vi "Splitter Manager UI.vi"(8 "error in (no error)":errorcluster, 11 "QD VI":refnum<vi>) -> (0 "error out":errorcluster)   [LabVIEW 2017]
uses:
  Splitter Info.ctl
panel:
  in  "Type Selector":enum32{"Splitters", "Panes"}(radio) caption="Radio Buttons"
  in  "Splitters":T1[](array[typedef])
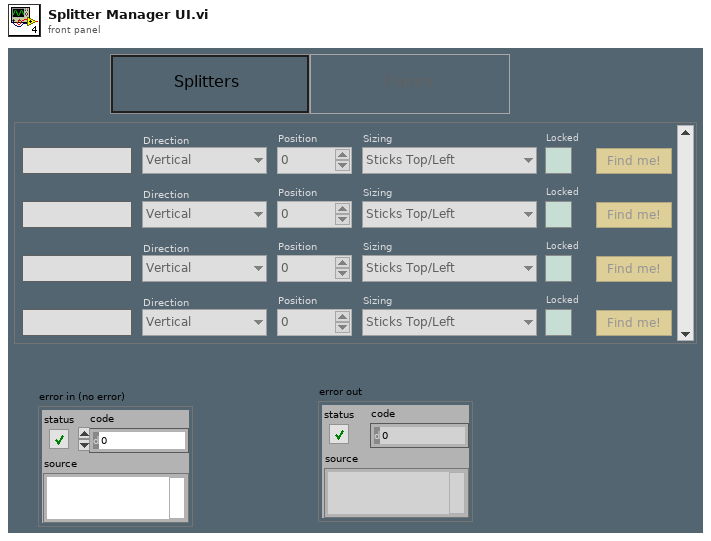
[diagram p1: front panel]
types:
  T1 = typedef "Splitter Info.ctl" = cluster{"Label":string, "Position":i32, "Sizing":enum16{"Sticks Top/Left", "Sticks Bottom/Right", "Proportional"}, "Locked":bool, "Highlight":bool, "Direction":enum16{"Vertical", "Horizontal"}}
  T2 = enum16{"Sticks Top/Left", "Sticks Bottom/Right", "Proportional"}
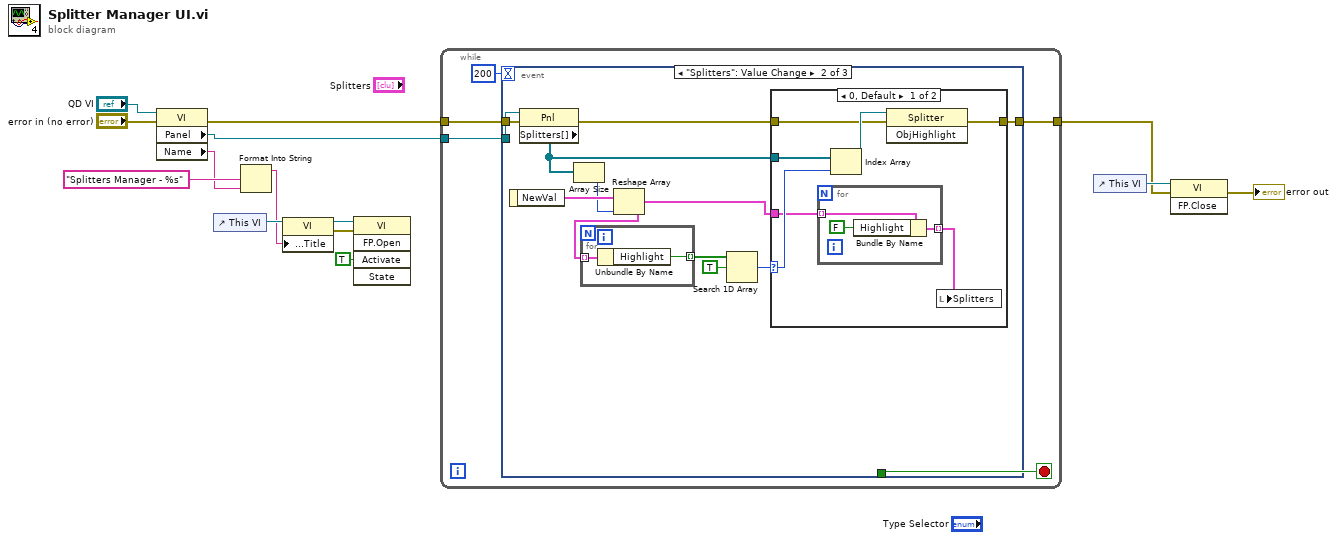
[diagram p0: block diagram]
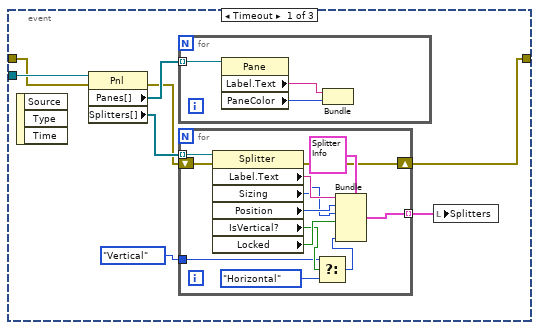
[diagram p2: hidden frame]
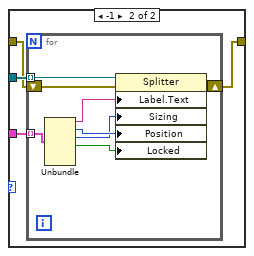
[diagram p3: hidden frame]
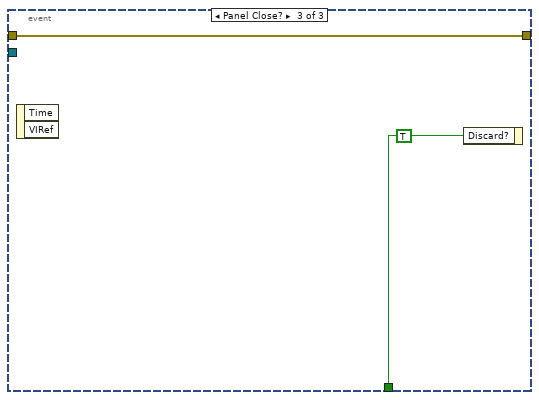
[diagram p4: hidden frame]
diagram:
  n1 = property class="VI"(reference="QD VI", error in="error in (no error)") -> (error out=w11:errorcluster, "Panel"=w12:refnum<vi>, "Name"=w5:string)  [unwired: 1 out]
  n2 = control-ref of="This VI"() -> (w7:refnum<vi>)
  n3 = Format Into String(format string="Splitters Manager - %s", w5) -> (resulting string=w4:string)  [unwired: 2 in, 1 out]
  n4 = property class="VI"(reference=w7, "Front Panel.Title"=w4) -> (reference out=w3:refnum<vi>, error out=w2:errorcluster)  [unwired: 1 in]
  n5 = invoke class="VI" method="FP.Open"(reference=w3, error in=w2, "Activate"=TRUE ("Activate?")) -> ()  [unwired: 2 in, 5 out]
  n6 = while {
    tunnel: w12 -> [w19]
    tunnel: w11 -> [w18]
    tunnel: [w16] -> w9
    stop <- w17 stop-if-true
    n7 = event shown="[1] \"Splitters\": Value Change" {
      selector: _ -> [_ _ _]
      dyn-events: _ -> [_ _ _]
      timeout: 200 -> [_ _ _]
      tunnel: w19 -> [w27 w54 _]
      tunnel: w18 -> [w26 w48 w79]
      tunnel: [_ _ w80] -> w17
      tunnel: [w21 w49 w79] -> w16
      event Timeout {
        n8 = event-data() -> ()  [unwired: 1 in, 3 out]
        n9 = property class="Pnl"(reference=w27, error in=w26) -> (error out=w20:errorcluster, "Panes[]"=w25:refnum<vi>[], "Splitters[]"=w24:refnum<vi>[])  [unwired: 1 out]
        n10 = for {
          tunnel: w25 -> [w43] mode=indexing
          n11 = property class="Pane"(reference=w43) -> ("Label.Text"=w42:string, "PaneColor"=w41:u32)  [unwired: 1 in, 2 out]
          n12 = Bundle("Label.Text"=w42, "PaneColor"=w41) -> ()  [unwired: 1 in, 1 out]
        }
        n13 = for {
          tunnel: w24 -> [w40] mode=indexing
          tunnel: [w36] -> w23 mode=indexing
          tunnel: enum16{"Vertical", "Horizontal"}."Vertical" -> [w32]
          shift-right: [w29] -> w21
          shift-left: w20 -> [w28]
          n14 = property class="Splitter"(reference=w40, error in=w28) -> (error out=w29:errorcluster, "Label.Text"=w39:string, "Sizing"=w34:T2, "Position"=w35:i32, "IsVertical?"=w33:bool, "Locked"=w38:bool)  [unwired: 1 out]
          n15 = Select(t=w32, s=w33, f=enum16{"Vertical", "Horizontal"}."Horizontal") -> (s? t:f=w31:enum16{"Vertical", "Horizontal"})
          n16 = Bundle(cluster=T1 {"Label"="", "Position"=0, "Sizing"=enum."Sticks Top/Left", "Locked"=FALSE, "Highlight"=FALSE, "Direction"=enum."Vertical"} ("output cluster"), "Label"=w39, "Position"=w35, "Sizing"=w34, "Locked"=w38, "Direction"=w31) -> (w36:T1)  [unwired: 1 in]
        }
        n17 = local write "Splitters"(w23) -> ()
      }
      event "Splitters": Value Change {
        n18 = event-data() -> ("NewVal"=w46:T1[])  [unwired: 1 in]
        n19 = property class="Pnl"(reference=w54, error in=w48) -> (error out=w53:errorcluster, "Splitters[]"=w47:refnum<vi>[])  [unwired: 1 out]
        n20 = Array Size(array=w47) -> (size(s)=w45:i32)
        n21 = Reshape Array(w46, w45) -> (w44:T1[])
        n22 = for {
          tunnel: w44 -> [w78] mode=indexing
          tunnel: [w77] -> w52 mode=indexing
          n23 = Unbundle By Name(w78) -> ("Highlight"=w77:bool)
        }
        n24 = Search 1D Array(1D array=w52, element=TRUE) -> (index of element=w50:i32)  [unwired: 1 in]
        n25 = case shown="0, Default" w50 {
          selector: w50 -> [w60 _]
          tunnel: w47 -> [w61 w68]
          tunnel: w53 -> [w55 w67]
          tunnel: w44 -> [w58 w66]
          tunnel: [w56 w65] -> w49
          frame 0, Default {
            n26 = for {
              tunnel: w58 -> [w63] mode=indexing
              tunnel: [w62] -> w57 mode=indexing
              n27 = Bundle By Name(cluster=w63, "Highlight"=FALSE) -> (w62:T1)
            }
            n28 = Index Array(array=w61, index=w60) -> (element=w59:refnum<vi>)
            n29 = invoke class="Splitter" method="ObjHighlight"(reference=w59, error in=w55) -> (error out=w56:errorcluster)  [unwired: 1 in, 2 out]
            n30 = local write "Splitters"(w57) -> ()
          }
          frame -1 {
            n31 = for {
              tunnel: w68 -> [w76] mode=indexing
              tunnel: w66 -> [w70] mode=indexing
              shift-right: [w69] -> w65
              shift-left: w67 -> [w75]
              n32 = Unbundle(w70) -> ("Label"=w74:string, "Position"=w73:i32, "Sizing"=w72:T2, "Locked"=w71:bool)  [unwired: 2 out]
              n33 = property class="Splitter"(reference=w76, error in=w75, "Label.Text"=w74, "Sizing"=w72, "Position"=w73, "Locked"=w71) -> (error out=w69:errorcluster)  [unwired: 1 out]
            }
          }
        }
      }
      event Panel Close? {
        w80 = TRUE ("Discard?")
        n34 = event-data() -> ()  [unwired: 1 in, 2 out]
        n35 = event-data("Discard?"=w80) -> ()  [unwired: 1 in, 1 out]
      }
    }
  }
  n36 = control-ref of="This VI"() -> (w10:refnum<vi>)
  n37 = invoke class="VI" method="FP.Close"(reference=w10, error in=w9) -> (error out=→"error out":errorcluster)  [unwired: 1 in, 2 out]
